vi "Append.vi"(6 "deadline":T1={"mode"=enum."Relative", "deadline (ms)"=30000}, 8 "error in (no error)":errorcluster, 10 "data":u8[](array[numeric]), 11 "Generic Download Controller in":refnum<class "Generic Download Controller.lvclass">) -> (0 "error out":errorcluster, 3 "Generic Download Controller out":refnum<class "Generic Download Controller.lvclass">)   [LabVIEW 2020, in "NI_SFTP.lvlib" / "Generic Download Controller.lvclass"]
uses:
  <vilib>/net/SFTP/API/Support/Download/Generic/Generic Download Controller.lvclass
  <vilib>/Utility/Deadline/Deadline.ctl
  <vilib>/Utility/Deadline/Mode.ctl
  <vilib>/Utility/Deadline/NI_Deadline.lvlib
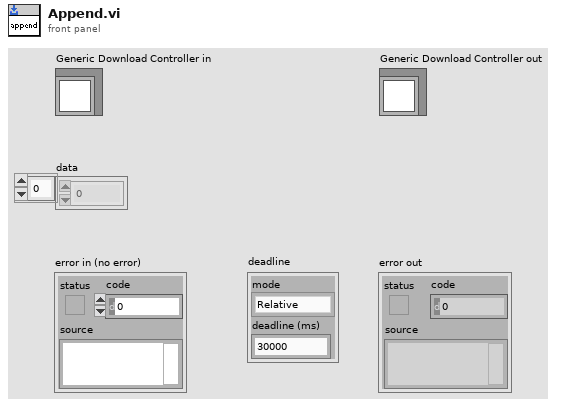
[diagram p1: front panel]
types:
  T1 = typedef "NI_Deadline.lvlib/Deadline.ctl" = cluster{"mode":T2, "deadline (ms)":u32}
  T2 = typedef "NI_Deadline.lvlib/Mode.ctl" = enum16{"Relative", "Use deadline", "Wait forever", "Nonblocking", "N/A"}
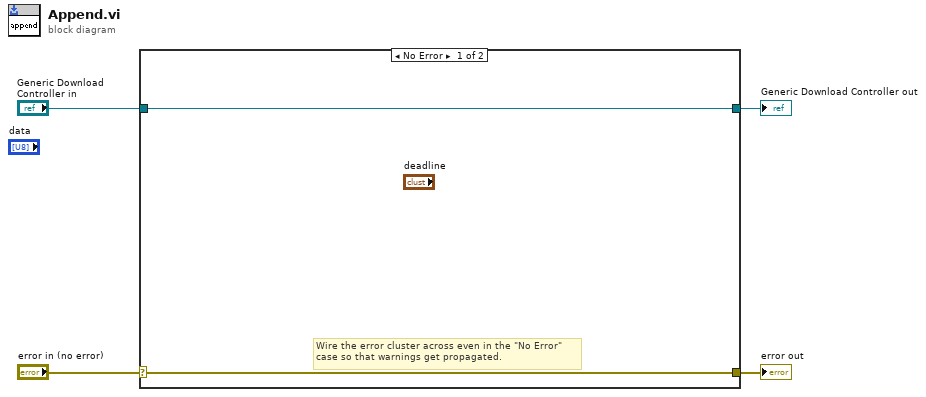
[diagram p0: block diagram]
diagram:
  n1 = case shown="No Error" "error in (no error)" {
    selector: "error in (no error)" -> [w5 w8]
    tunnel: [w5 w8] -> w3
    tunnel: [w6 w7] -> w1
    tunnel: "Generic Download Controller in" -> [w6 w7]
    frame No Error {
      # "Wire the error cluster across even in the \"No Error\"\ncase so that warnings get propagated."
    }
    frame Error {
    }
  }
  "error out" <- w3
  "Generic Download Controller out" <- w1
